vi "WriteSound.vi"() -> ()   [LabVIEW 2015]
uses:
  <vilib>/sound2/lvsound2.llb/Sampling Mode.ctl
  <vilib>/sound2/lvsound2.llb/Sound File Info (path).vi
  <vilib>/sound2/lvsound2.llb/Sound File Read Open.vi
  <vilib>/sound2/lvsound2.llb/Sound File Read (DBL).vi
  <vilib>/sound2/lvsound2.llb/Sound Output Set Volume (Single).vi
  <vilib>/sound2/lvsound2.llb/Sound Output Write (DBL).vi
panel:
  in  "stop":bool
  out "Loop Index":i32
  in  "volume":dbl=100.0
  in  "device ID":u32
  in  "number of samples/ch":i32=100000
  in  "path":path
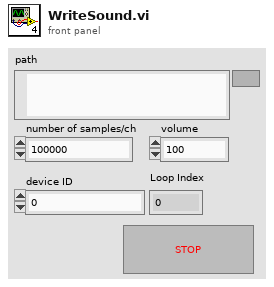
[diagram p1: front panel]
types:
  T1 = typedef "Sampling Mode.ctl" = i32
  T2 = typedef "Sound Data Format.ctl" = cluster{"sample rate (S/s)":dbl, "number of channels":i32, "bits per sample":i32}
  T3 = typedef "Sound File Refnum.ctl" = refnum<file>
  T4 = typedef "Sound Output Task ID.ctl" = u32
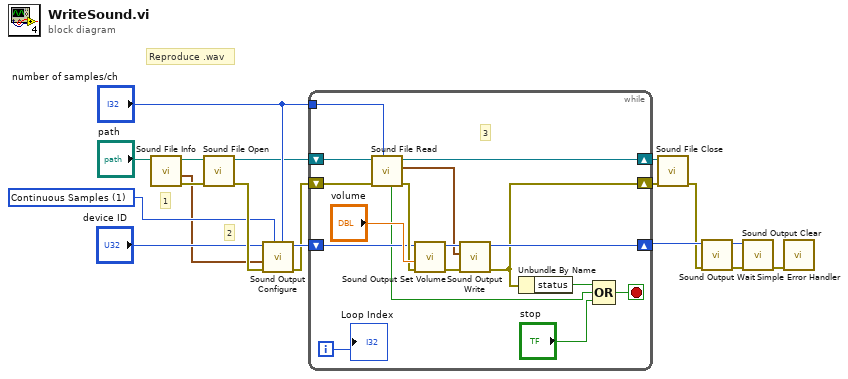
[diagram p0: block diagram]
diagram:
  w14 = T1 1 items=["Finite Samples", "Continuous Samples"] ("sample mode")
  # "Reproduce .wav"
  # "1"
  # "2"
  n1 = call-poly <vilib>:"Sound File Info.vi"("path"="path") -> ("error out"=w16:errorcluster, "sound format"=w12:T2, "path out"=w17:path)  [unwired: 7 in, 1 out]
  n2 = call-poly <vilib>:"Sound File Open.vi"("error in (no error)"=w16, "path"=w17) -> ("error out"=w15:errorcluster, "sound file refnum"=w9:T3)  [unwired: 8 in]
  n3 = call <vilib>:"Sound Output Configure.vi"("number of samples/ch"="number of samples/ch", "sample mode"=w14, "error in (no error)"=w15, "sound format"=w12, "device ID"="device ID") -> ("error out"=w8:errorcluster, "task ID"=w11:T4)  [unwired: 5 in]
  n4 = while {
    shift-right: [w25] -> w5
    shift-left: w11 -> [w30]
    tunnel: "number of samples/ch" -> [w35]
    shift-right: [w26] -> w6
    shift-left: w9 -> [w34]
    shift-right: [w24] -> w7
    shift-left: w8 -> [w33]
    i -> [w23]
    stop <- w19 stop-if-true
    # "3"
    n5 = call-poly <vilib>:"Sound File Read.vi"("number of samples/ch (-1: all)"=w35, "error in (no error)"=w33, "sound file refnum"=w34) -> ("error out"=w31:errorcluster, "data"=w27:waveform(dbl)[], "sound file refnum out"=w26:T3, "end of file?"=w21:bool)  [unwired: 4 in, 1 out]
    n6 = call-poly <vilib>:"Sound Output Set Volume.vi"("error in (no error)"=w31, "volume"="volume", "task ID"=w30) -> ("error out"=w29:errorcluster, "task ID out"=w28:T4)  [unwired: 7 in]
    n7 = call-poly <vilib>:"Sound Output Write.vi"("error in (no error)"=w29, "data"=w27, "task ID"=w28) -> ("error out"=w24:errorcluster, "task ID out"=w25:T4)  [unwired: 7 in]
    n8 = Unbundle By Name(w24) -> ("status"=w22:bool)
    n9 = Compound Arithmetic op=OR(w22, w21, "stop") -> (w19:bool)
    "Loop Index" <- w23
  }
  n10 = call <vilib>:"Sound File Close.vi"("error in (no error)"=w7, "sound file refnum"=w6) -> ("error out"=w4:errorcluster)  [unwired: 9 in]
  n11 = call <vilib>:"Sound Output Wait.vi"("error in (no error)"=w4, "task ID"=w5) -> ("error out"=w3:errorcluster, "task ID out"=w2:T4)  [unwired: 8 in]
  n12 = call <vilib>:"Sound Output Clear.vi"("error in (no error)"=w3, "task ID"=w2) -> ("error out"=w1:errorcluster)  [unwired: 9 in]
  n13 = call <vilib>:"Simple Error Handler.vi"("error in (no error)"=w1) -> ()  [unwired: 4 in, 5 out]
